vi "Compute Split Range.vi"(9 "limit size":i32, 10 "length":i32, 11 "start":i32) -> (2 "terminal length":i32, 3 "initial length":i32)   [LabVIEW 2020, in "NI_Bytestream.lvlib" / "Bytestream.lvclass"]
uses:
  <vilib>/Array/Bytestream/Bytestream.lvclass
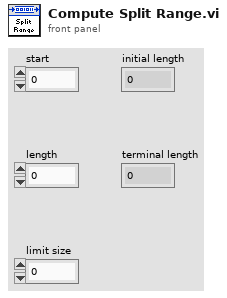
[diagram p1: front panel]
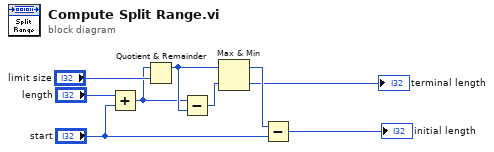
[diagram p0: block diagram]
diagram:
  n1 = Add(x="length", y="start") -> (x+y=w4:i32)
  n2 = Quotient & Remainder(x=w4, y="limit size") -> (x-y*floor(x/y)=w6:i32)  [unwired: 1 out]
  n3 = Subtract(x=w4, y=w6) -> (x-y=w7:i32)
  n4 = Max & Min(x=w6, y=w7) -> (max(x,y)=w8:i32, min(x,y)=→"terminal length":i32)
  n5 = Subtract(x=w8, y="start") -> (x-y=→"initial length":i32)
